vi "ParseVectorFile.ParseSVG.vi"(8 "error in (no error)":errorcluster, 10 "Path":path, 11 "ParseVectorFile in":refnum<class "ParseVectorFile.lvclass">) -> (0 "error out":errorcluster, 3 "ParseVectorFile out":refnum<class "ParseVectorFile.lvclass">)   [LabVIEW 2019, in "ParseVectorFile.lvclass"]
uses:
  ParseVectorFile.lvclass
  ParseVectorFile.lvclass/ParseVectorFile.ctl
panel:
  out "Total":u32
  out "Get SVG Objects":u32
  out "Path Fact":u32
  out "Rect Fact":u32
  out "Image Fact":u32
  out "Circe Fact":u32
  # "Reentrant allocation"
  # "118\n114\n117"
  # "99\n158\n128\n142\n147\n161"
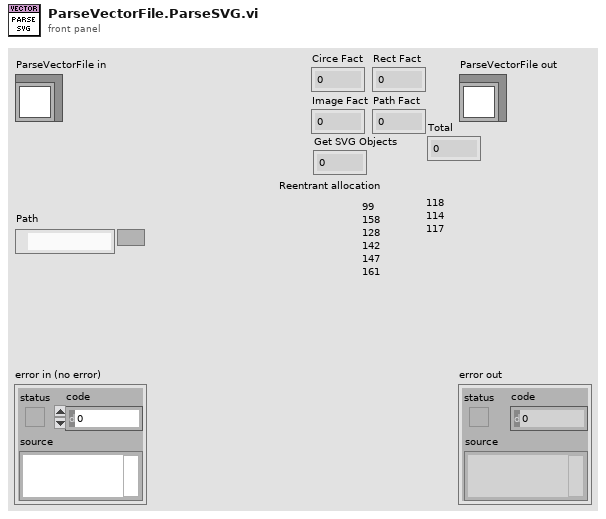
[diagram p1: front panel]
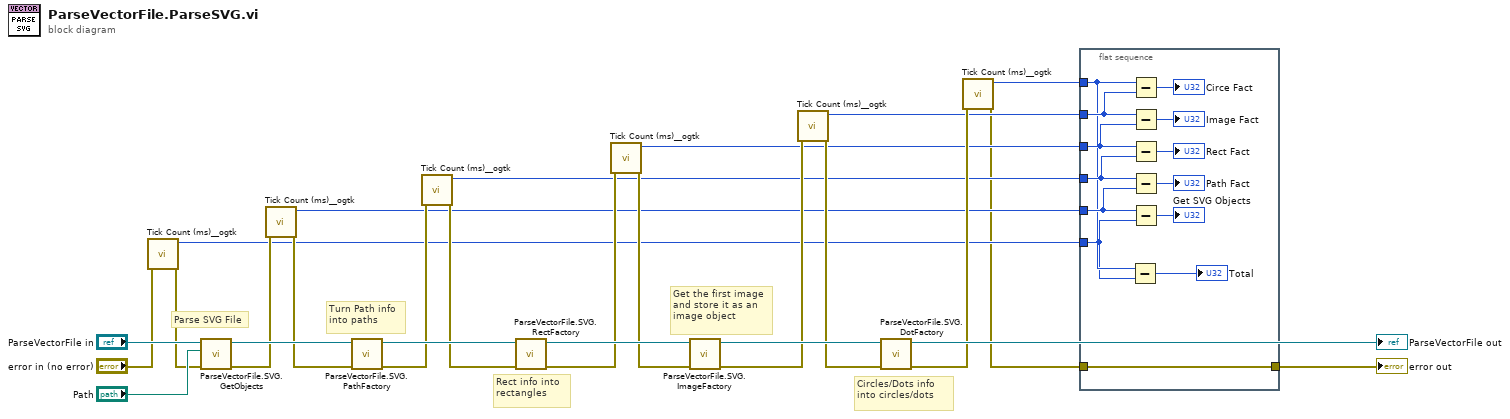
[diagram p0: block diagram]
diagram:
  # "Circles/Dots info into circles/dots"
  # "Get the first image and store it as an image object"
  # "Rect info into rectangles"
  # "Turn Path info into paths"
  # "Parse SVG File"
  n1 = call <userlib>:"Tick Count (ms)__ogtk.vi"("error in (no error)"="error in (no error)") -> ("error out"=w18:errorcluster, "millisecond timer value"=w3:u32)  [unwired: 9 in]
  n2 = call "ParseVectorFile.SVG.GetObjects.vi"("error in (no error)"=w18, "Path"="Path", "ParseVectorFile in"="ParseVectorFile in") -> ("error out"=w17:errorcluster, "ParseVectorFile out"=w24:refnum<class "ParseVectorFile.lvclass">)  [unwired: 7 in]
  n3 = call <userlib>:"Tick Count (ms)__ogtk.vi"("error in (no error)"=w17) -> ("error out"=w16:errorcluster, "millisecond timer value"=w4:u32)  [unwired: 9 in]
  n4 = call "ParseVectorFile.SVG.PathFactory.vi"("error in (no error)"=w16, "ParseVectorFile in"=w24) -> ("error out"=w15:errorcluster, "ParseVectorFile out"=w23:refnum<class "ParseVectorFile.lvclass">)  [unwired: 8 in]
  n5 = call <userlib>:"Tick Count (ms)__ogtk.vi"("error in (no error)"=w15) -> ("error out"=w14:errorcluster, "millisecond timer value"=w5:u32)  [unwired: 9 in]
  n6 = call "ParseVectorFile.SVG.RectFactory.vi"("error in (no error)"=w14, "ParseVectorFile in"=w23) -> ("error out"=w13:errorcluster, "ParseVectorFile out"=w22:refnum<class "ParseVectorFile.lvclass">)  [unwired: 8 in]
  n7 = call <userlib>:"Tick Count (ms)__ogtk.vi"("error in (no error)"=w13) -> ("error out"=w12:errorcluster, "millisecond timer value"=w6:u32)  [unwired: 9 in]
  n8 = call "ParseVectorFile.SVG.ImageFactory.vi"("error in (no error)"=w12, "ParseVectorFile in"=w22) -> ("error out"=w11:errorcluster, "ParseVectorFile out"=w21:refnum<class "ParseVectorFile.lvclass">)  [unwired: 8 in]
  n9 = call <userlib>:"Tick Count (ms)__ogtk.vi"("error in (no error)"=w11) -> ("error out"=w10:errorcluster, "millisecond timer value"=w7:u32)  [unwired: 9 in]
  n10 = call "ParseVectorFile.SVG.DotFactory.vi"("error in (no error)"=w10, "ParseVectorFile in"=w21) -> ("error out"=w9:errorcluster, "ParseVectorFile out"=→"ParseVectorFile out":refnum<class "ParseVectorFile.lvclass">)  [unwired: 8 in]
  n11 = call <userlib>:"Tick Count (ms)__ogtk.vi"("error in (no error)"=w9) -> ("error out"=w2:errorcluster, "millisecond timer value"=w8:u32)  [unwired: 9 in]
  n12 = flat-sequence {
    tunnel: w8 -> [w29]
    tunnel: w7 -> [w38]
    tunnel: w6 -> [w37]
    tunnel: w5 -> [w36]
    tunnel: w4 -> [w35]
    tunnel: w3 -> [w28]
    tunnel: w2 -> [w39]
    tunnel: [w39] -> w1
    frame #0 {
      n13 = Subtract(x=w29, y=w28) -> (x-y=→"Total":u32)
      n14 = Subtract(x=w29, y=w38) -> (x-y=→"Circe Fact":u32)
      n15 = Subtract(x=w38, y=w37) -> (x-y=→"Image Fact":u32)
      n16 = Subtract(x=w37, y=w36) -> (x-y=→"Rect Fact":u32)
      n17 = Subtract(x=w36, y=w35) -> (x-y=→"Path Fact":u32)
      n18 = Subtract(x=w35, y=w28) -> (x-y=→"Get SVG Objects":u32)
    }
  }
  "error out" <- w1
